vi "Stop Core.vi"(10 "final error code":i32, 11 "ZenGage v3.0 UI in":refnum<class "ZenGage v3.0 UI.lvclass">) -> (3 "ZenGage v3.0 UI out":refnum<class "ZenGage v3.0 UI.lvclass">)   [LabVIEW 2019, in "ZenGage v3.0 UI.lvclass"]
doc: "(<B>Filename</B>: Actor Framework.lvlib:Actor.lvclass:Stop Core.vi)\n\nDefines what the actor does before it stops. Use the <B>final error code</B> input to determine whether the actor shut down in response to an error.\n\nBy default, this method does nothing. A descendant class may override it to define behavior, such as shutting down any processes the actor initiated in its override of the Actor Core method."
uses:
  ZenGage v3.0 UI.lvclass
  <vilib>/ActorFramework/Actor/Actor.lvclass
  <vilib>/event_ctls.llb/usereventprio.ctl
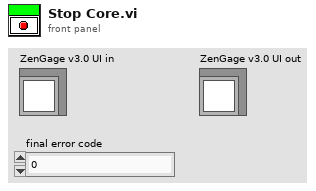
[diagram p1: front panel]
types:
  T1 = typedef "usereventprio.ctl" = enum32{"high priority", "normal priority"}
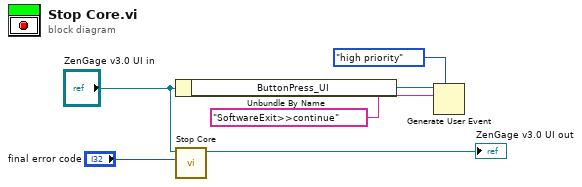
[diagram p0: block diagram]
diagram:
  n1 = Unbundle By Name("ZenGage v3.0 UI in") -> ("ButtonPress_UI"=w3:refnum<user-event>)
  n2 = call-parent "Stop Core.vi"("final error code"="final error code", "Actor in"="ZenGage v3.0 UI in") -> ("Actor out"=→"ZenGage v3.0 UI out":refnum<class "ZenGage v3.0 UI.lvclass">)  [unwired: 9 in]
  n3 = Generate User Event(priority (normal)=usereventprio."high priority", user event=w3, event data cluster="SoftwareExit>>continue" ("Functionality name")) -> ()  [unwired: 1 in, 2 out]
